vi "test_db.vi"() -> ()   [LabVIEW 2014]
uses:
  <vilib>/addons/database/Connection.llb/DB Tools Open Connec (String).vi
  <vilib>/addons/database/Connection.llb/Conn Execute.vi
  <vilib>/addons/database/Recordset.llb/Rec Fetch Integer Data (R).vi
  <vilib>/addons/database/Recordset.llb/Rec Destroy - Connection.vi
  <vilib>/addons/database/_DB Variant To Data/Database Variant To Data.xnode
  <vilib>/addons/database/NI_Database_API.lvlib
  FT_HMI.llb/TYPE_DEF_PUMP_RESULTS.ctl
panel:
  out "Nbre de lignes 3":i32
  in  "stop":bool
  in  "CHANGE VALUE":bool
  in  "flag_print_ok":i32=2
  out "appended array":string[](array[string])
  out "resulting string":string
  in  "N° de serie":string
  out "element 2":string
  out "element":string
  out "columns":string[](array[string])
  out "Array":string[][](array[string])
  out "data":variant[][](array[variant])
  out "Nbre de lignes 5":i32
  out "Nbre de lignes 4":i32
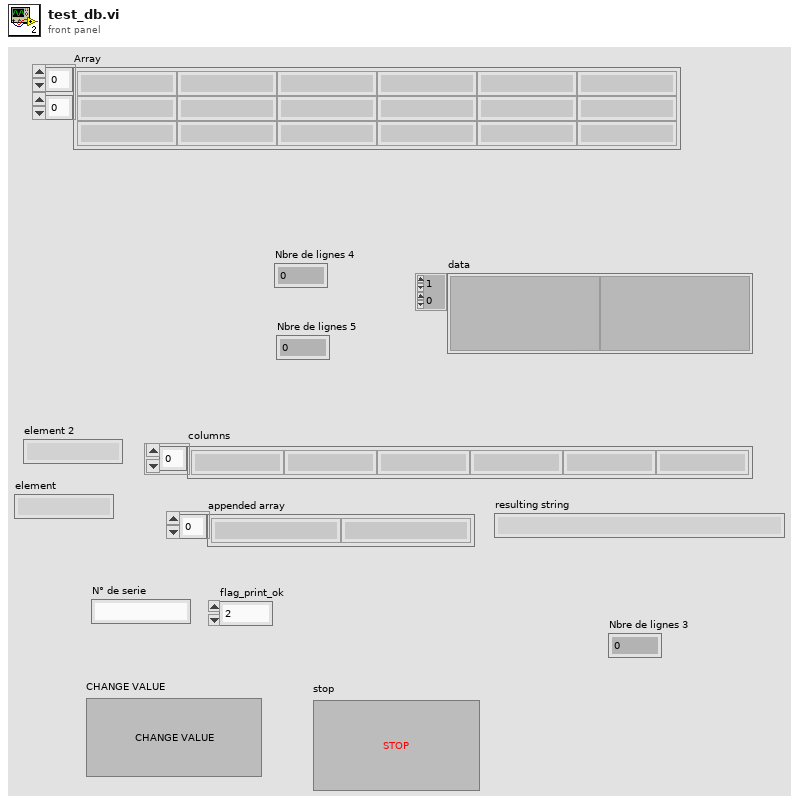
[diagram p1: front panel]
types:
  T1 = typedef "NI_Database_API.lvlib/Conn ObjectReference.ctl" = refnum<k1>
  T2 = typedef "TYPE_DEF_PUMP_RESULTS.ctl" = cluster{"ID_resultat":string, "No d'article":string, "Designation":string, "No OF":string, "No de serie":string, "Horodatage":string, "Test HT":i8, "Aspiration [m]":sgl, "Perte asp [mbar]":sgl, "Etancheite [mbar]":sgl, "Debit max [l/h]":sgl, "Débit travail [l/h]":sgl, "Perte de charge pression [bar]":sgl, "Perte de charge aspiration [bar] ":sgl, "Courant max [mA]":sgl, "By-pass":i8, "Pression max [bar]":sgl, "Perte pression [mbar]":sgl, "Pump status":bool, "status HT":i8, "status aspiration":i8, "status perte aspiration":i8, "status etancheite":i8, "status Q max":i8, "status Q t ravail":i8, "status I max":i8, "status by-pass":i8, "status P max":i8, "status Perte pression":i8, "flag_print":string}
  T3 = typedef "NI_Database_API.lvlib/Rec ObjectReference.ctl" = refnum<k1>
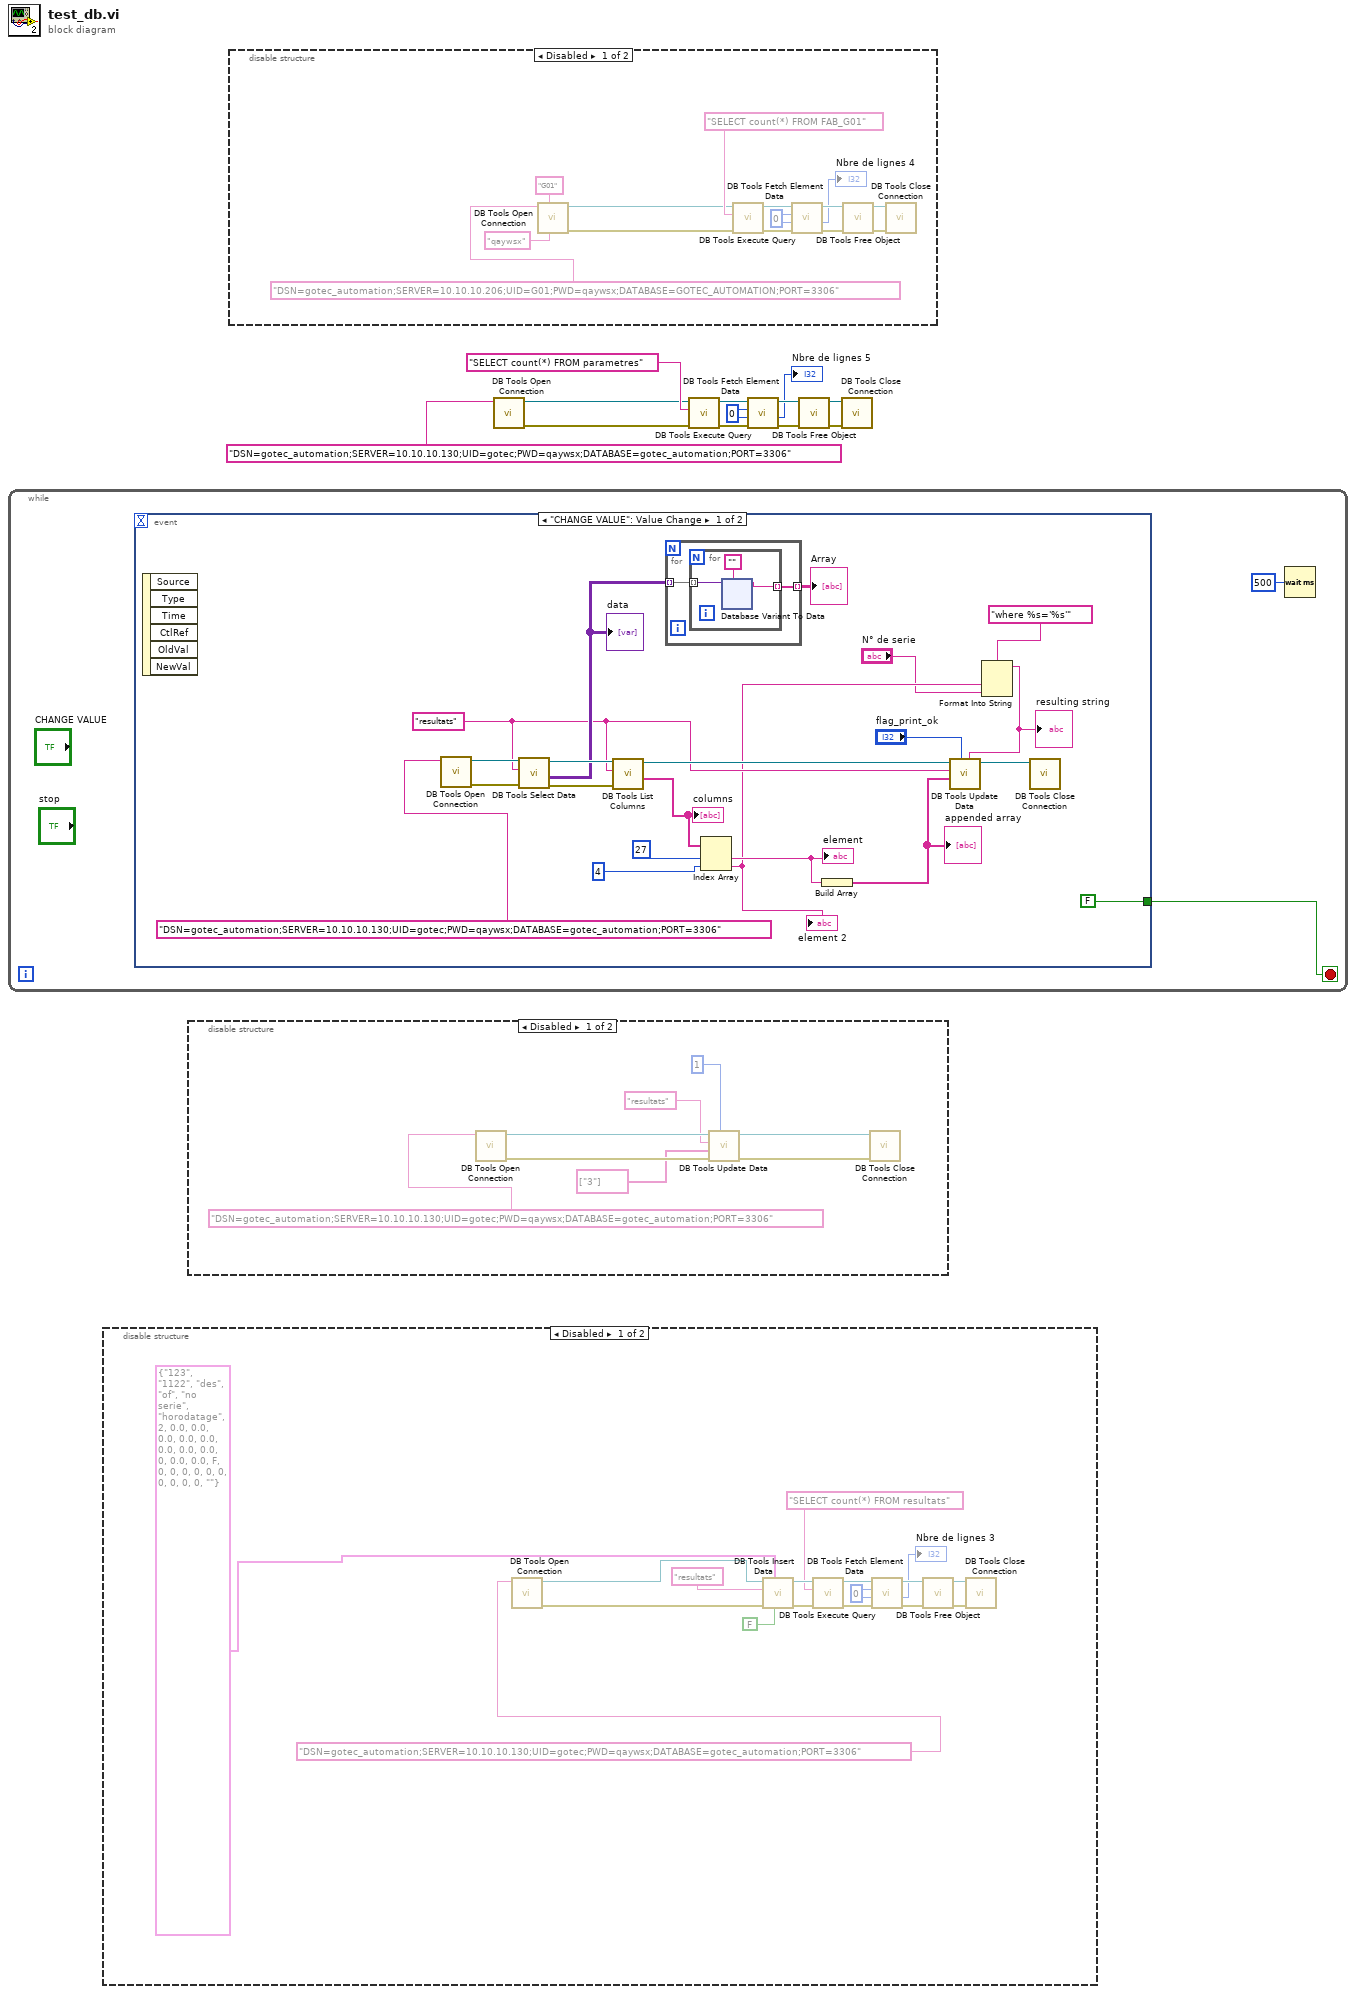
[diagram p0: block diagram]
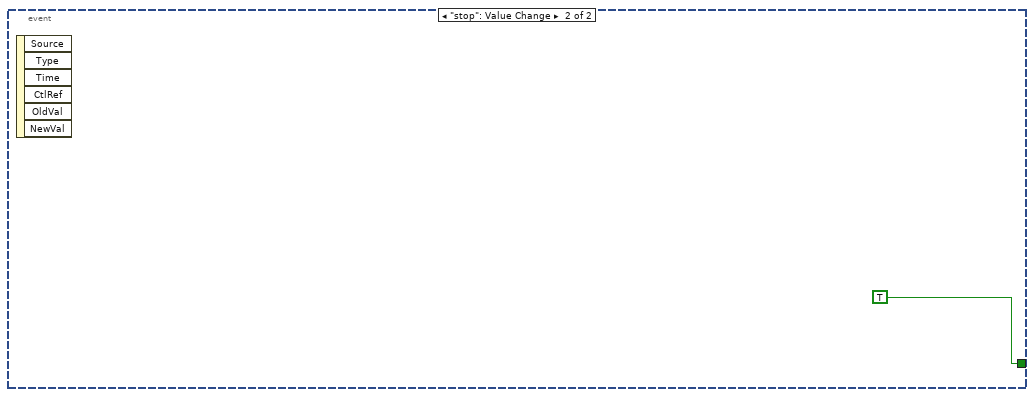
[diagram p3: hidden frame]
diagram:
  w5 = 0
  n1 = while {
    stop <- w13 stop-if-true
    n2 = event shown="[0] \"CHANGE VALUE\": Value Change" {
      selector: _ -> [_ _]
      dyn-events: _ -> [_ _]
      timeout: _ -> [_ _]
      tunnel: [FALSE TRUE] -> w13
      event "CHANGE VALUE": Value Change {
        w24 = "resultats" ("SQL query")
        n3 = event-data() -> ()  [unwired: 1 in, 6 out]
        n4 = call-poly <vilib>:"DB Tools Open Connection.vi"("connection information"="DSN=gotec_automation;SERVER=10.10.10.130;UID=gotec;PWD=qaywsx;DATABASE=gotec_automation;PORT=3306") -> ("error out"=w33:errorcluster, "connection reference"=w34:T1)  [unwired: 7 in]
        n5 = call <vilib>:"DB Tools Select Data.vi"("error in (no error)"=w33, "table"=w24, "connection reference"=w34) -> ("error out"=w31:errorcluster, "data"=w30:variant[][], "connection reference out"=w32:T1)  [unwired: 3 in]
        "data" <- w30
        n6 = call <vilib>:"DB Tools List Columns.vi"("error in (no error)"=w31, "table"=w24, "connection reference"=w32) -> ("columns"=w28:string[], "connection reference out"=w26:T1)  [unwired: 1 in, 2 out]
        "columns" <- w28
        n7 = for {
          tunnel: w30 -> [w37] mode=indexing
          tunnel: [w36] -> w29 mode=indexing
          n8 = for {
            tunnel: w37 -> [w39] mode=indexing
            tunnel: [w38] -> w36 mode=indexing
            n9 = xnode "Database Variant To Data"("database variant"=w39, "type"="") -> ("data"=w38:string)  [unwired: 1 in, 1 out]
          }
        }
        "Array" <- w29
        n10 = Index Array(array=w28, index #1=27 ("index"), index #2=4 ("index")) -> (element #1=w23:string, element #2=w19:string)
        "element" <- w23
        "element 2" <- w19
        n11 = Build Array(w23) -> (w22:string[])
        "appended array" <- w22
        n12 = Format Into String(format string="where %s='%s'", w19, "N° de serie") -> (resulting string=w17:string)  [unwired: 2 in, 1 out]
        "resulting string" <- w17
        n13 = call <vilib>:"DB Tools Update Data.vi"("condition"=w17, "data"="flag_print_ok", "columns"=w22, "table"=w24, "connection reference"=w26) -> ("connection reference out"=w25:T1)  [unwired: 5 in, 1 out]
        n14 = call <vilib>:"DB Tools Close Connection.vi"("connection reference"=w25) -> ()  [unwired: 6 in, 1 out]
      }
      event "stop": Value Change {
        n15 = event-data() -> ()  [unwired: 1 in, 6 out]
      }
    }
    n16 = Wait (ms)(milliseconds to wait=u32 500) -> ()  [unwired: 1 out]
  }
  n17 = disable-structure shown="Disabled" {
    frame Disabled {
      w77 = 0
      n18 = call-poly <vilib>:"DB Tools Open Connection.vi"("connection information"="DSN=gotec_automation;SERVER=10.10.10.130;UID=gotec;PWD=qaywsx;DATABASE=gotec_automation;PORT=3306") -> ("error out"=w89:errorcluster, "connection reference"=w90:T1)  [unwired: 7 in]
      n19 = call <vilib>:"DB Tools Insert Data.vi"("flatten cluster? (F)"=FALSE, "data"=T2 {"ID_resultat"="123", "No d'article"="1122", "Designation"="des", "No OF"="of", "No de serie"="no serie", "Horodatage"="horodatage", "Test HT"=2, "Aspiration [m]"=0.0, "Perte asp [mbar]"=0.0, "Etancheite [mbar]"=0.0, "Debit max [l/h]"=0.0, "Débit travail [l/h]"=0.0, "Perte de charge pression [bar]"=0.0, "Perte de charge aspiration [bar] "=0.0, "Courant max [mA]"=0.0, "By-pass"=0, "Pression max [bar]"=0.0, "Perte pression [mbar]"=0.0, "Pump status"=FALSE, "status HT"=0, "status aspiration"=0, "status perte aspiration"=0, "status etancheite"=0, "status Q max"=0, "status Q t ravail"=0, "status I max"=0, "status by-pass"=0, "status P max"=0, "status Perte pression"=0, "flag_print"=""} ("Pump_Results"), "error in (no error)"=w89, "table"="resultats", "connection reference"=w90) -> ("error out"=w80:errorcluster, "connection reference out"=w81:T1)  [unwired: 5 in]
      n20 = call-poly <vilib>:"DB Tools Execute Query.vi"("error in (no error)"=w80, "SQL query"="SELECT count(*) FROM resultats", "connection reference"=w81) -> ("error out"=w86:errorcluster, "recordset reference"=w82:T3)  [unwired: 5 in]
      n21 = call-poly <vilib>:"DB Tools Fetch Element Data.vi"("error in (no error)"=w86, "type"=w77, "column index"=w77, "recordset reference"=w82) -> ("error out"=w85:errorcluster, "data"=→"Nbre de lignes 3":i32, "recordset reference out"=w83:T3)  [unwired: 3 in]
      n22 = call-poly <vilib>:"DB Tools Free Object.vi"("error in (no error)"=w85, "recordset reference"=w83) -> ("error out"=w79:errorcluster, "connection reference"=w84:T1)  [unwired: 8 in]
      n23 = call <vilib>:"DB Tools Close Connection.vi"("error in (no error)"=w79, "connection reference"=w84) -> ()  [unwired: 5 in, 1 out]
    }
    frame Enabled {
    }
  }
  n24 = disable-structure shown="Disabled" {
    frame Disabled {
      n25 = call-poly <vilib>:"DB Tools Open Connection.vi"("connection information"="DSN=gotec_automation;SERVER=10.10.10.130;UID=gotec;PWD=qaywsx;DATABASE=gotec_automation;PORT=3306") -> ("error out"=w95:errorcluster, "connection reference"=w97:T1)  [unwired: 7 in]
      n26 = call <vilib>:"DB Tools Update Data.vi"("data"=1, "error in (no error)"=w95, "columns"=string[] ["3"], "table"="resultats" ("SQL query"), "connection reference"=w97) -> ("error out"=w93:errorcluster, "connection reference out"=w94:T1)  [unwired: 5 in]
      n27 = call <vilib>:"DB Tools Close Connection.vi"("error in (no error)"=w93, "connection reference"=w94) -> ()  [unwired: 5 in, 1 out]
    }
    frame Enabled {
    }
  }
  n28 = disable-structure shown="Disabled" {
    frame Disabled {
      w103 = 0
      n29 = call-poly <vilib>:"DB Tools Open Connection.vi"("password"="qaywsx", "userID"="G01", "connection information"="DSN=gotec_automation;SERVER=10.10.10.206;UID=G01;PWD=qaywsx;DATABASE=GOTEC_AUTOMATION;PORT=3306") -> ("error out"=w99:errorcluster, "connection reference"=w100:T1)  [unwired: 5 in]
      n30 = call-poly <vilib>:"DB Tools Execute Query.vi"("error in (no error)"=w99, "SQL query"="SELECT count(*) FROM FAB_G01", "connection reference"=w100) -> ("error out"=w110:errorcluster, "recordset reference"=w106:T3)  [unwired: 5 in]
      n31 = call-poly <vilib>:"DB Tools Fetch Element Data.vi"("error in (no error)"=w110, "type"=w103, "column index"=w103, "recordset reference"=w106) -> ("error out"=w109:errorcluster, "data"=→"Nbre de lignes 4":i32, "recordset reference out"=w107:T3)  [unwired: 3 in]
      n32 = call-poly <vilib>:"DB Tools Free Object.vi"("error in (no error)"=w109, "recordset reference"=w107) -> ("error out"=w105:errorcluster, "connection reference"=w108:T1)  [unwired: 8 in]
      n33 = call <vilib>:"DB Tools Close Connection.vi"("error in (no error)"=w105, "connection reference"=w108) -> ()  [unwired: 5 in, 1 out]
    }
    frame Enabled {
    }
  }
  n34 = call-poly <vilib>:"DB Tools Open Connection.vi"("connection information"="DSN=gotec_automation;SERVER=10.10.10.130;UID=gotec;PWD=qaywsx;DATABASE=gotec_automation;PORT=3306") -> ("error out"=w1:errorcluster, "connection reference"=w2:T1)  [unwired: 7 in]
  n35 = call-poly <vilib>:"DB Tools Execute Query.vi"("error in (no error)"=w1, "SQL query"="SELECT count(*) FROM parametres", "connection reference"=w2) -> ("error out"=w12:errorcluster, "recordset reference"=w8:T3)  [unwired: 5 in]
  n36 = call-poly <vilib>:"DB Tools Fetch Element Data.vi"("error in (no error)"=w12, "type"=w5, "column index"=w5, "recordset reference"=w8) -> ("error out"=w11:errorcluster, "data"=→"Nbre de lignes 5":i32, "recordset reference out"=w9:T3)  [unwired: 3 in]
  n37 = call-poly <vilib>:"DB Tools Free Object.vi"("error in (no error)"=w11, "recordset reference"=w9) -> ("error out"=w7:errorcluster, "connection reference"=w10:T1)  [unwired: 8 in]
  n38 = call <vilib>:"DB Tools Close Connection.vi"("error in (no error)"=w7, "connection reference"=w10) -> ()  [unwired: 5 in, 1 out]
